vi "Test 02.vi"() -> ()   [LabVIEW 2021]
uses:
  <vilib>/Platform/TimedLoop/XDataNode/timing_clust.ctl
  <vilib>/Platform/TimedLoop/XDataNode/nitl_modes.ctl
  <vilib>/Platform/TimedLoop/XDataNode/wakeup.ctl
  <vilib>/MakerHub/LINX/Public/Utilities/Open Serial.vi
  <vilib>/Utility/file.llb/Write Delimited Spreadsheet (DBL).vi
  <vilib>/platform/TimedLoop/XDataNode/XDataNode.xnode
  <vilib>/Platform/TimedLoop/XDataNode/XDNodeRunTimeDep.lvlib
  <vilib>/MakerHub/LINX/LMH-LINX.lvlib
panel:
  out "dt":dbl
  out "Overrun":bool
  in  "Serial Port":refnum<visa-resource-name>
  in  "Stop Button":bool
  out "theta":dbl(graph)=0.10008950000019468
  in  "Motor command":dbl
  in  "Reset":bool
  in  "Kp":dbl=15.0
  out "omega":cluster{"y_dot":dbl, "Output":dbl}(graph)
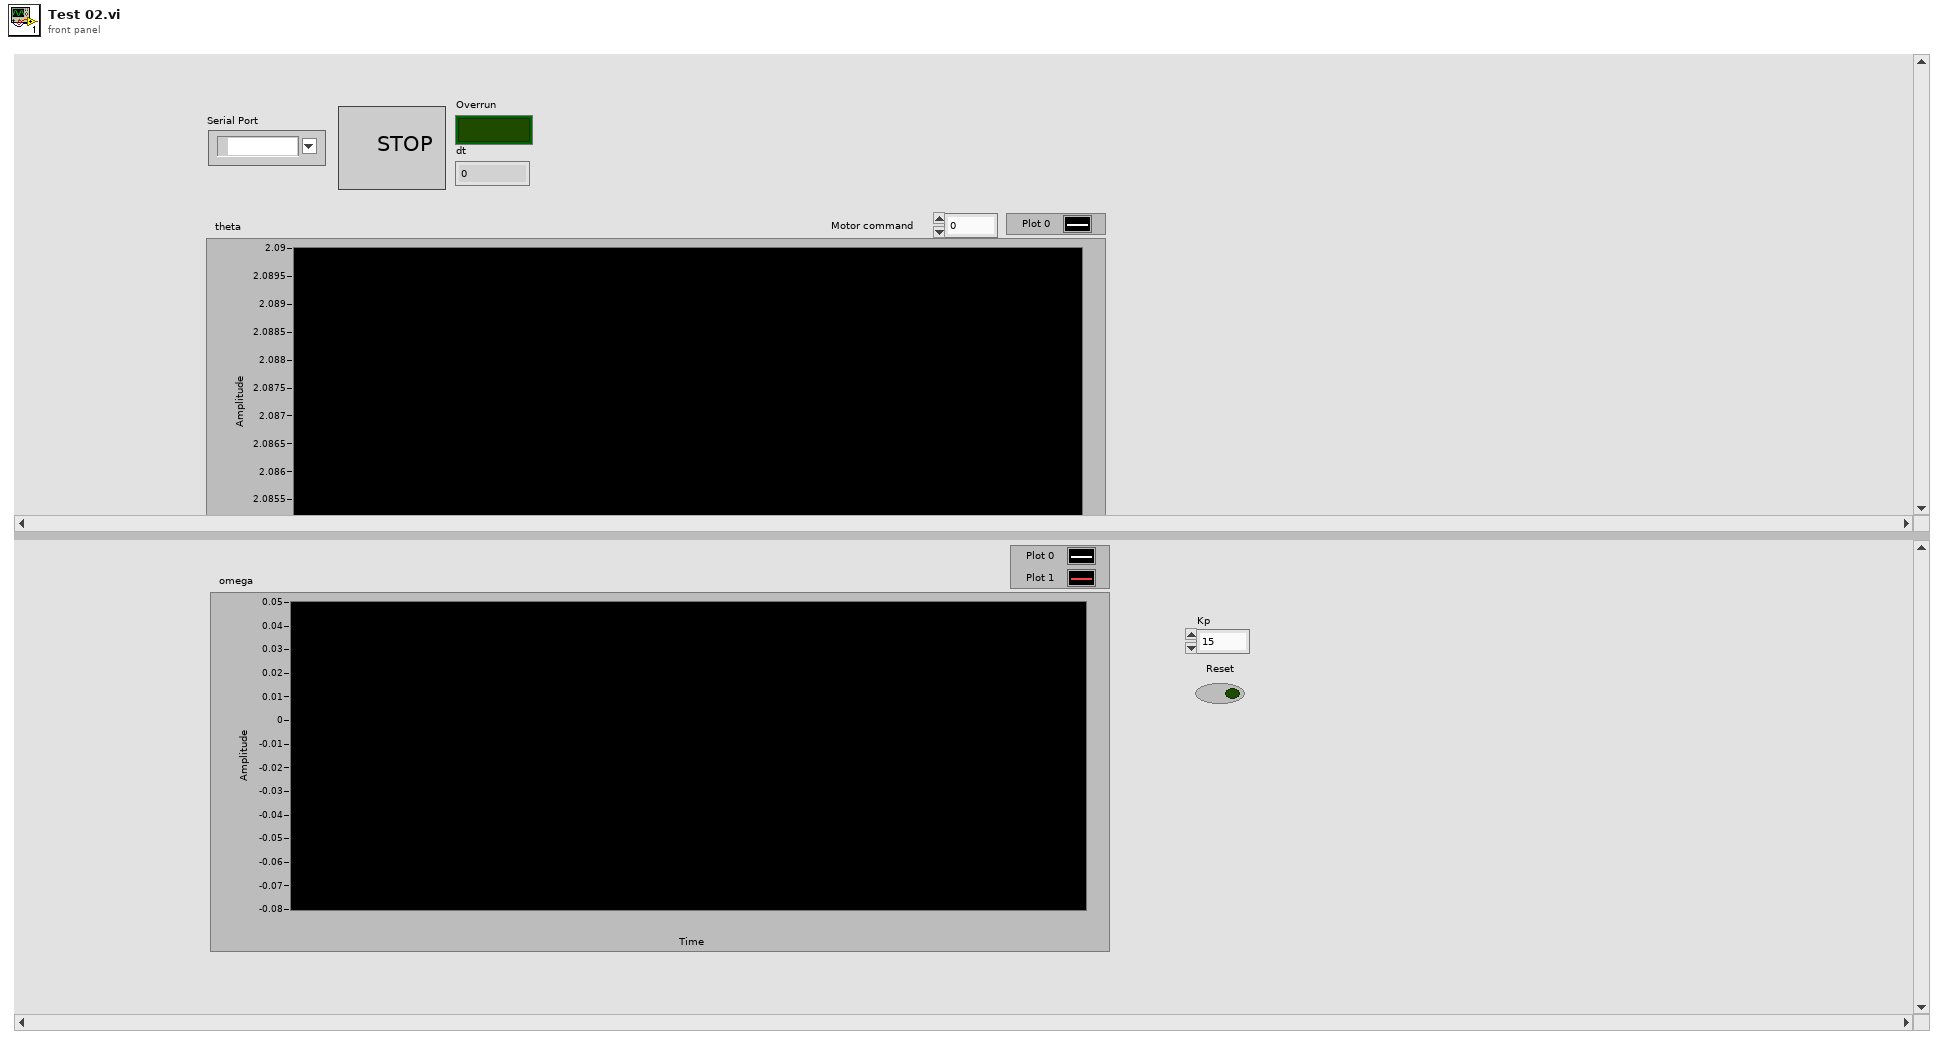
[diagram p1: front panel]
types:
  T1 = typedef "XDNodeRunTimeDep.lvlib/timing_clust.ctl" = cluster{"Expected End [f-1]":u64, "Actual End [f-1]":u64, "Finished Late? [f-1]":bool, "Expected End [i-1]":u64, "Actual End [i-1]":u64, "Finished Late? [i-1]":bool, "Expected Start [i]":u64, "Actual Start [i]":u64, "Expected Start [f]":u64, "Actual Start [f]":u64, "Source Name":string, "Structure Name":string, "Period":i64, "Deadline":i64, "Offset":i64, "Start":i64, "Priority":i32, "Timeout":i32, "Mode":T2, "Wakeup Reason":T3, "Error":errorcluster, "Source Type":string, "Secondary Source Type":string, "Global End Time":u64, "Global Start Time":u64, "Frame Duration":u64, "Iteration Duration":u64, "Assigned CPU":i32, "I/O Scan Engine Mode":u32}
  T2 = typedef "XDNodeRunTimeDep.lvlib/nitl_modes.ctl" = enum32{"No Change", "Process missed periods, maintain original phase", "Discard missed periods, maintain original phase", "Process missed periods, ignore original phase", "Discard missed periods, ignore original phase"}
  T3 = typedef "XDNodeRunTimeDep.lvlib/wakeup.ctl" = enum32{"Normal", "Aborted", "Asynchronous wakeup", "Timing source error", "Timed loop error", "Timeout"}
  T4 = typedef "LMH-LINX.lvlib/LINX Ref.ctl" = cluster{"IO":T5, "Interface":T6, "LINX Device Config":T7}
  T5 = typedef "LMH-LINX.lvlib/Platform.ctl" = enum16{"Remote", "Local"}
  T6 = typedef "LMH-LINX.lvlib/Interface.ctl" = enum16{"Serial", "TCP"}
  T7 = typedef "LMH-LINX.lvlib/Device.lvlib/LINX Device Config.ctl" = cluster{"Interface":T6, "COM Port":refnum<visa-resource-name>, "TCP Configuration":T8, "Device Family":u8, "Device ID":u8, "Device Name":string, "TCP Ref":refnum<k5>, "Channels":T9}
  T8 = typedef "LMH-LINX.lvlib/Device.lvlib/TCP Config.ctl" = cluster{"IP Address":string, "Port":u16}
  T9 = typedef "LMH-LINX.lvlib/Channels.ctl" = cluster{"DI":u8[], "DO":u8[], "AI":u8[], "AO":u8[], "PWM":u8[], "QE":u8[], "UART":u8[], "I2C 2":u8[], "SPI":u8[], "CAN":u8[], "Servo":u8[], "AI Ref (V)":dbl, "AI Resolution (Bits)":u8, "AO Ref (V)":dbl, "AO Resolution (Bits)":u8}
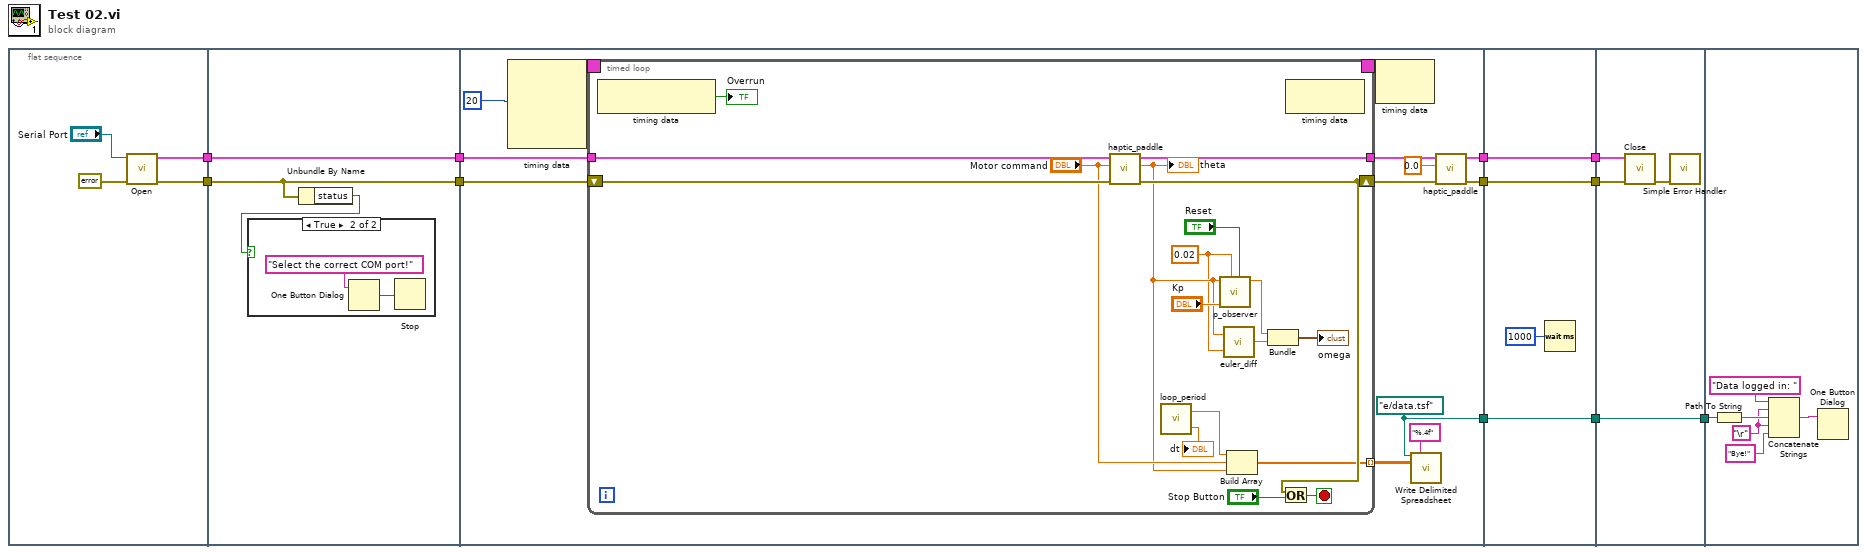
[diagram p0: block diagram]
diagram:
  n1 = flat-sequence {
    tunnel: [w13] -> w7
    tunnel: [w12] -> w5
    tunnel: w7 -> [w18]
    tunnel: [w18] -> w6
    tunnel: w5 -> [w17]
    tunnel: [w17] -> w4
    tunnel: [w28] -> w10
    tunnel: [w27] -> w8
    tunnel: w6 -> [w26]
    tunnel: w4 -> [w25]
    tunnel: [w21] -> w3
    tunnel: [w61] -> w11
    tunnel: w10 -> [w61]
    tunnel: [w60] -> w9
    tunnel: w8 -> [w60]
    tunnel: w3 -> [w59]
    tunnel: [w59] -> w2
    tunnel: w11 -> [w65]
    tunnel: w9 -> [w64]
    tunnel: w2 -> [w63]
    tunnel: [w63] -> w1
    tunnel: w1 -> [w72]
    frame #0 {
      n2 = call-poly <vilib>:"Open.vi"("Error In"=errorcluster {"status"=FALSE, "code"=0, "source"=""}, "Serial Port"="Serial Port") -> ("Error Out"=w12:errorcluster, "LINX Resource"=w13:T4)  [unwired: 7 in, 1 out]
    }
    frame #1 {
      n3 = Unbundle By Name(w17) -> ("status"=w16:bool)
      n4 = case shown="True" w16 {
        frame False {
        }
        frame True {
          n5 = One Button Dialog(message="Select the correct COM port!") -> (true=w19:bool)  [unwired: 1 in]
          n6 = Stop(stop? (T)=w19) -> ()
        }
      }
    }
    frame #2 {
      w21 = path "e:/data.tsf" ("file path (dialog if empty)")
      n7 = node-c288(i64 20 ("Period")) -> (w33:T1)  [unwired: 3 in]
      n8 = timed-loop {
        tunnel: w26 -> [w47]
        tunnel: [w49] -> w30
        shift-right: [w48] -> w29
        shift-left: w25 -> [w46]
        timing: w33 -> [_]
        timing-out: [_] -> w32
        tunnel: [w44] -> w23 mode=indexing
        stop <- w51 stop-if-true
        w37 = 0.02 ("dt")
        n9 = node-c288() -> (→"Overrun":bool)  [unwired: 1 in]
        n10 = call "haptic_paddle.vi"("Error In"=w46, "PWM Input"="Motor command", "LINX Resource In"=w47) -> ("Error Out"=w48:errorcluster, "Angular Output"=w38:dbl, "LINX Resource Out"=w49:T4)  [unwired: 6 in]
        "theta" <- w38
        n11 = call "loop_period.vi"() -> ("dt"=→"dt":dbl, "t"=w43:dbl)  [unwired: 3 in]
        n12 = call "p_observer.vi"("y"=w38, "Kp"="Kp", "dt"=w37, "Reset"="Reset") -> ("y_dot"=w35:dbl)  [unwired: 6 in]
        n13 = call "euler_diff.vi"("dt"=w37, "Input"=w38) -> ("Output"=w36:dbl)
        n14 = Build Array(w43, "Motor command", w38) -> (w44:dbl[])
        n15 = Bundle("y_dot"=w35, "Output"=w36) -> (→"omega":cluster{"y_dot":dbl, "Output":dbl})  [unwired: 1 in]
        n16 = Or(x=w48, y="Stop Button") -> (x .or. y?=w51:bool)
        n17 = node-c288() -> ()  [unwired: 1 in, 1 out]
      }
      n18 = node-c288(w32) -> ()  [unwired: 1 out]
      n19 = call-poly <vilib>:"Write Delimited Spreadsheet.vi"("file path (dialog if empty)"=w21, "format (%.3f)"="%.4f", "2D data"=w23) -> ()  [unwired: 11 in, 2 out]
      n20 = call "haptic_paddle.vi"("Error In"=w29, "PWM Input"=0.0, "LINX Resource In"=w30) -> ("Error Out"=w27:errorcluster, "LINX Resource Out"=w28:T4)  [unwired: 6 in, 1 out]
    }
    frame #3 {
      n21 = Wait (ms)(milliseconds to wait=u32 1000) -> ()  [unwired: 1 out]
    }
    frame #4 {
      n22 = call <vilib>:"Close.vi"("Error In"=w64, "LINX Resource"=w65) -> ("Error Out"=w66:errorcluster)  [unwired: 9 in]
      n23 = call <vilib>:"Simple Error Handler.vi"("error in (no error)"=w66) -> ()  [unwired: 4 in, 5 out]
    }
    frame #5 {
      w67 = "\r"
      n24 = Path To String(path=w72) -> (string=w71:string)
      n25 = Concatenate Strings("Data logged in: " ("message"), w67, w71, w67, "Bye!" ("string")) -> (w69:string)
      n26 = One Button Dialog(message=w69) -> ()  [unwired: 1 in, 1 out]
    }
  }
